vi "trójkąt.vi"() -> ()   [LabVIEW 2020]
panel:
  out "TRÓJKĄT":waveform(dbl)(graph)
  in  "Częstotliwość":dbl(knob)=478.47412109375 scale=0.0..1000.0
  in  "Amplituda":dbl(knob)=0.7659562800187257 scale=0.0..1.0 scale format="%.1f"
  in  "Wzmocnienie\n     szumu":dbl(slide)=0.01020408163265306 scale=0.0..1.0
  in  "Typ sygnału":u16(ring)=4 items=["szum ", "zewnętrzny", "sinus", "prostokąt", "trójkąt"]
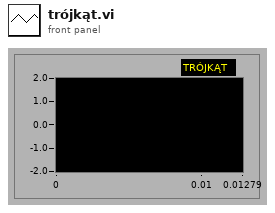
[diagram p1: front panel]
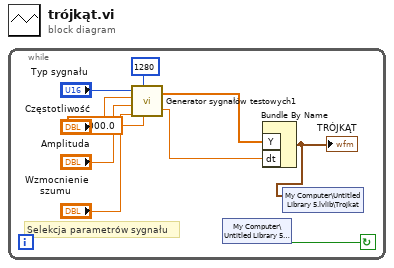
[diagram p0: block diagram]
diagram:
  n1 = while {
    stop <- w2 continue-if-true
    # "Selekcja parametrów sygnału"
    n2 = call "Generator sygnałów testowych1.vi"("częstość pobierania\nserii próbek"=100000.0 ("częstość pobierania\nserii próbek"), "liczba punktów\n      (1024)"=1280, "amplituda  szumów"="Wzmocnienie\n     szumu", "amplituda"="Amplituda", "częstotliwość"="Częstotliwość", "typ sygnału"="Typ sygnału") -> ("czas pobierania\nserii próbek"=w3:dbl, "Sygnał wyjściowy"=w4:dbl[])
    n3 = shared-variable "My Computer\\Untitled Library 5.lvlib\\Stop"() -> (w2:bool)  [unwired: 1 in, 1 out]
    n4 = Bundle By Name("Y"=w4, "dt"=w3) -> (w1:waveform(dbl))  [unwired: 1 in]
    "TRÓJKĄT" <- w1
    n5 = shared-variable "My Computer\\Untitled Library 5.lvlib\\Trojkat"(w1) -> ()  [unwired: 1 in, 1 out]
  }
